vi "Update Steering Motor Angle State_Frame.vi"(8 "error in (no error)":errorcluster, 10 "ccw motor angle state (rad)":dbl, 11 "wheel in":refnum<class "NI_Robotics_Wheel.lvclass">) -> (0 "error out":errorcluster, 1 "failed?":bool, 3 "wheel out":refnum<class "NI_Robotics_Wheel.lvclass">)   [LabVIEW 2017, in "NI_Robotics_Wheel.lvclass"]
uses:
  <vilib>/robotics/Steering/Wheel/NI_Robotics_Wheel.lvclass
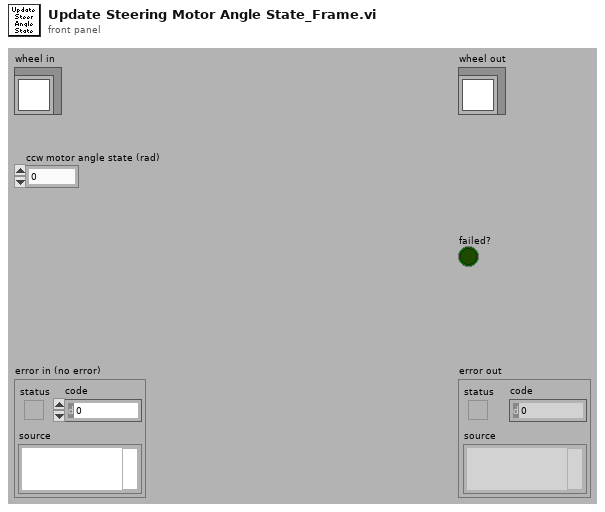
[diagram p1: front panel]
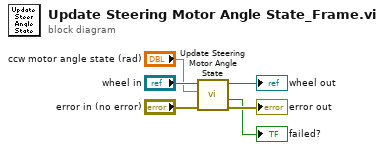
[diagram p0: block diagram]
diagram:
  n1 = call-dynamic "Update Steering Motor Angle State.vi"("error in (no error)"="error in (no error)", "ccw motor angle state (rad)"="ccw motor angle state (rad)", "wheel in"="wheel in") -> ("error out"=→"error out":errorcluster, "failed?"=→"failed?":bool, "wheel out"=→"wheel out":refnum<class "NI_Robotics_Wheel.lvclass">)  [unwired: 6 in]
